vi "RT Config - Dual RT Sweep.vi"(8 "error in (no error)":errorcluster, 11 "1553 Unit Test in":refnum<class "Remote Terminal.lvclass">) -> (0 "error out":errorcluster, 3 "1553 Unit Test out":refnum<class "Remote Terminal.lvclass">)   [LabVIEW 2020, in "Unit Tests.lvlib" / "Remote Terminal.lvclass"]
uses:
  Remote Terminal.lvclass
  Remote Terminal.lvclass/Remote Terminal.ctl
  Remote Terminal/TypeDefs/RT Command Config.ctl
  Frames & Messages/TypeDefs/Command Type.ctl
  Frames & Messages/TypeDefs/Command SubAddress.ctl
  Frames & Messages/TypeDefs/Command Word Count.ctl
  Frames & Messages/TypeDefs/Simplified Parameter Data Table.ctl
  Frames & Messages/TypeDefs/Scaling Information.ctl
  Remote Terminal/TypeDefs/RT Configuration.ctl
  Remote Terminal/TypeDefs/RT-RT Timeout.ctl
  Remote Terminal/TypeDefs/Mode Code 17 Sync Configuration.ctl
  Remote Terminal/TypeDefs/RT Timetag Configuration.ctl
  Remote Terminal/Remote Terminal.lvclass
  C:/Users/MattJ/Desktop/git/bci-1553-labview-api/src/1553 SubComponent/1553 SubComponent.lvclass
  1553 Session/1553 Session.lvclass
  1553 Component/1553 Component.lvclass
  <vilib>/addons/_JKI Toolkits/Caraya/classes/Test/Test.lvclass
  BCI-1553 API.lvlib
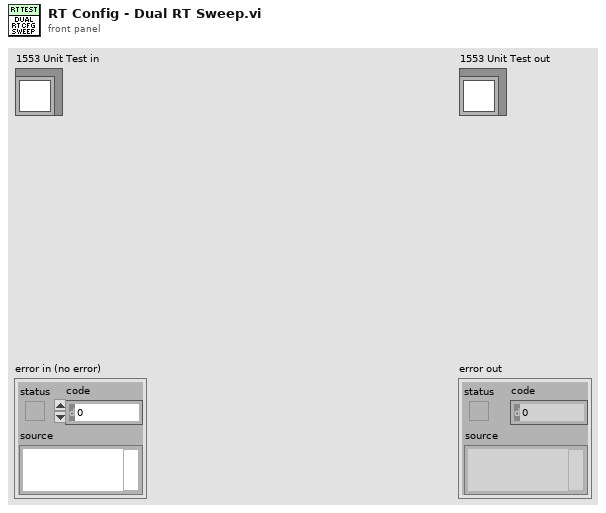
[diagram p1: front panel]
types:
  T1 = typedef "BCI-1553 API.lvlib/Simplified Parameter Data Table.ctl" = cluster{"Parameter Name":string, "Base Word":u16, "Scaling Info":T2}
  T2 = typedef "BCI-1553 API.lvlib/Scaling Information.ctl" = cluster{"Bit Offset":i32, "Bit Count":i32, "LSB Resolution":dbl, "2's Complement":bool, "Big Endian":bool, "Sign Bit":bool}
  T3 = typedef "BCI-1553 API.lvlib/Command SubAddress.ctl" = enum16{"Mode Code", "1", "2", "3", "4", "5", "6", "7", "8", "9", "10", "11", "12", "13", "14", "15", "16", "17", "18", "19", "20", "21", "22", "23", "24", "25", "26", "27", "28", "29", "30"}
  T4 = typedef "BCI-1553 API.lvlib/Command Type.ctl" = enum16{"Transmit", "Receive"}
  T5 = typedef "BCI-1553 API.lvlib/Remote Terminal.lvclass/RT Command Config.ctl" = cluster{"Command Type":T4, "SubAddress":T3, "Word Count\\Mode Code":T6, "Initial Data":u16[], "Data Fields":T1[]}
  T6 = typedef "BCI-1553 API.lvlib/Command Word Count.ctl" = enum16{"1", "2", "3", "4", "5", "6", "7", "8", "9", "10", "11", "12", "13", "14", "15", "16", "17", "18", "19", "20", "21", "22", "23", "24", "25", "26", "27", "28", "29", "30", "31", "32"}
  T7 = typedef "BCI-1553 API.lvlib/Remote Terminal.lvclass/RT Configuration.ctl" = cluster{"RT-RT Timeout":T8, "Inhibit Bus A":bool, "Inhibit Bus B":bool, "Broadcast CMD Invalid":bool, "UnDef MCs Invalid":bool, "Notice 2 Data Storage":bool, "SMCP":bool, "Temp RX Buffer":bool, "Alt BIT Enable":bool, "Auto Bus Shutdown":bool, "MC 16 SR Reset":bool, "MC 17 Sync":T9, "MC 8 Reset":bool, "Remote Terminal Timetag Config":T10}
  T8 = typedef "BCI-1553 API.lvlib/Remote Terminal.lvclass/RT-RT Timeout.ctl" = enum16{"57us", "62us", "100us", "180us"}
  T9 = typedef "BCI-1553 API.lvlib/Remote Terminal.lvclass/Mode Code 17 Sync Configuration.ctl" = enum16{"Sync if Bit 0 = 1", "Sync if Bit 0 = 0", "Sync Unconditionally"}
  T10 = typedef "BCI-1553 API.lvlib/Remote Terminal.lvclass/RT Timetag Configuration.ctl" = enum16{"Disabled", "2us", "4us", "8us", "16us", "32us", "64us"}
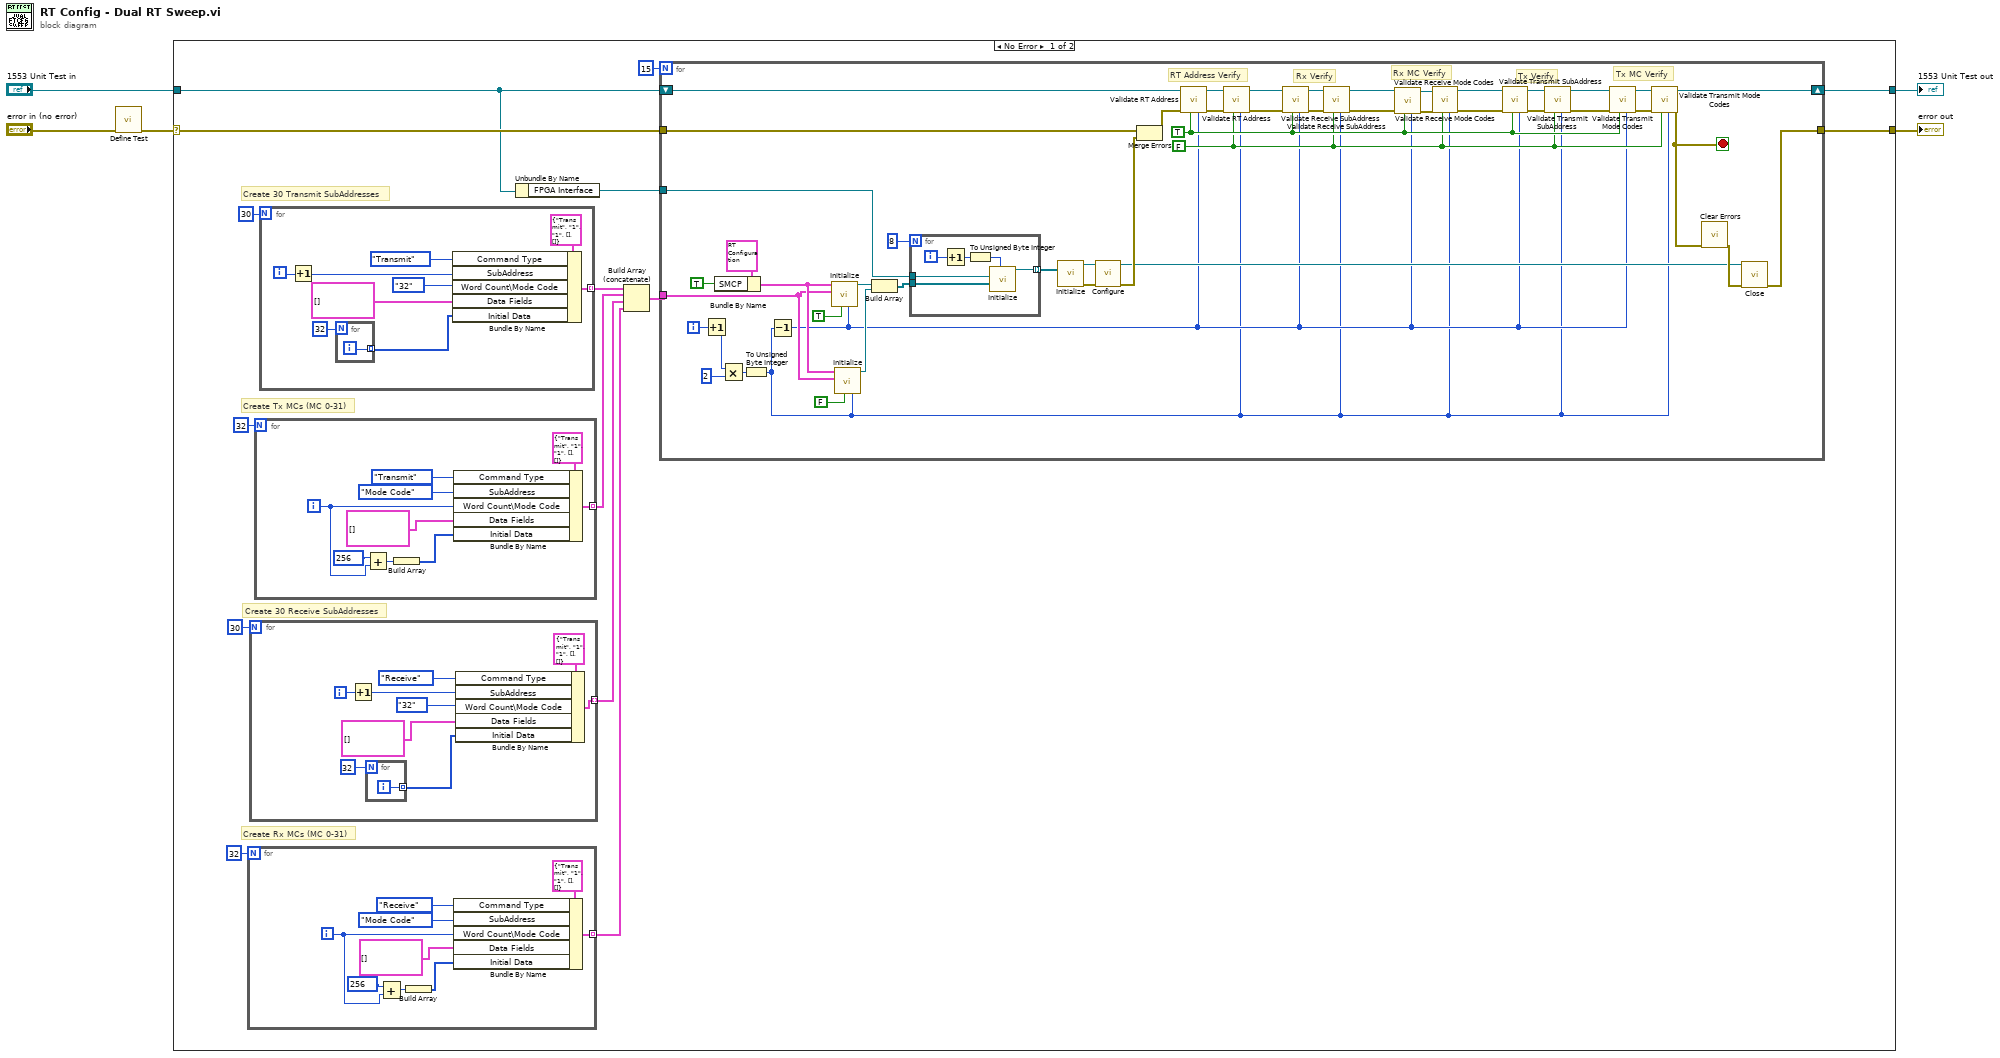
[diagram p0: block diagram]
diagram:
  n1 = call <vilib>:"Define Test.vi"("error in (no error)"="error in (no error)") -> ("error out"=w1:errorcluster)  [unwired: 9 in, 1 out]
  n2 = case shown="No Error" w1 {
    selector: w1 -> [w17 w115]
    tunnel: [w18 w115] -> w5
    tunnel: [w19 w114] -> w3
    tunnel: "1553 Unit Test in" -> [w16 w114]
    frame No Error {
      # "Create Rx MCs (MC 0-31)"
      # "Create Tx MCs (MC 0-31)"
      # "Create 30 Receive SubAddresses"
      # "Create 30 Transmit SubAddresses"
      n3 = for {
        N: 32 -> [_]
        tunnel: [w29] -> w7 mode=indexing
        i -> [w22]
        n4 = Add(x=256, y=w22) -> (x+y=w23:i32)
        n5 = Build Array(w23) -> (w25:i32[])
        n6 = Bundle By Name(cluster=T5 {"Command Type"=enum."Transmit", "SubAddress"=enum."1", "Word Count\\Mode Code"=enum."1", "Initial Data"=[], "Data Fields"=[]} ("RT Commands"), "Command Type"=Command_Type."Receive", "SubAddress"=Command_SubAddress."Mode Code", "Word Count\\Mode Code"=w22, "Data Fields"=T1[] [], "Initial Data"=w25) -> (w29:T5)
      }
      n7 = for {
        N: 30 -> [_]
        tunnel: [w47] -> w9 mode=indexing
        i -> [w42]
        n8 = Increment(x=w42) -> (x+1=w41:i32)
        n9 = for {
          N: 32 -> [_]
          tunnel: [w48] -> w43 mode=indexing
          i -> [w48]
        }
        n10 = Bundle By Name(cluster=T5 {"Command Type"=enum."Transmit", "SubAddress"=enum."1", "Word Count\\Mode Code"=enum."1", "Initial Data"=[], "Data Fields"=[]} ("RT Commands"), "Command Type"=Command_Type."Receive", "SubAddress"=w41, "Word Count\\Mode Code"=Command_Word_Count."32" ("Word Count\\Mode Code"), "Data Fields"=T1[] [], "Initial Data"=w43) -> (w47:T5)
      }
      n11 = for {
        N: 32 -> [_]
        tunnel: [w38] -> w10 mode=indexing
        i -> [w32]
        n12 = Add(x=256, y=w32) -> (x+y=w33:i32)
        n13 = Build Array(w33) -> (w31:i32[])
        n14 = Bundle By Name(cluster=T5 {"Command Type"=enum."Transmit", "SubAddress"=enum."1", "Word Count\\Mode Code"=enum."1", "Initial Data"=[], "Data Fields"=[]} ("RT Commands"), "Command Type"=Command_Type."Transmit", "SubAddress"=Command_SubAddress."Mode Code", "Word Count\\Mode Code"=w32, "Data Fields"=T1[] [], "Initial Data"=w31) -> (w38:T5)
      }
      n15 = for {
        N: 30 -> [_]
        tunnel: [w57] -> w12 mode=indexing
        i -> [w52]
        n16 = Increment(x=w52) -> (x+1=w51:i32)
        n17 = for {
          N: 32 -> [_]
          tunnel: [w58] -> w53 mode=indexing
          i -> [w58]
        }
        n18 = Bundle By Name(cluster=T5 {"Command Type"=enum."Transmit", "SubAddress"=enum."1", "Word Count\\Mode Code"=enum."1", "Initial Data"=[], "Data Fields"=[]} ("RT Commands"), "Command Type"=Command_Type."Transmit", "SubAddress"=w51, "Word Count\\Mode Code"=Command_Word_Count."32" ("Word Count\\Mode Code"), "Data Fields"=T1[] [], "Initial Data"=w53) -> (w57:T5)
      }
      n19 = Unbundle By Name(w16) -> ("FPGA Interface"=w15:refnum<class "FPGA Interface.lvclass">)
      n20 = Build Array (concatenate)(w12, w10, w9, w7) -> (w6:T5[])
      n21 = for {
        N: 15 -> [_]
        shift-right: [w74] -> w19
        shift-left: w16 -> [w97]
        tunnel: [w83] -> w18
        tunnel: w17 -> [w92]
        tunnel: w6 -> [w82]
        tunnel: w15 -> [w81]
        i -> [w104]
        stop <- w70 stop-if-true
        w72 = FALSE ("RT 1?")
        w73 = TRUE ("RT 1?")
        # "Tx MC Verify"
        # "Rx MC Verify"
        # "RT Address Verify"
        # "Rx Verify"
        # "Tx Verify"
        n22 = Increment(x=w104) -> (x+1=w88:i32)
        n23 = Bundle By Name(cluster=T7 {"RT-RT Timeout"=enum."57us", "Inhibit Bus A"=FALSE, "Inhibit Bus B"=FALSE, "Broadcast CMD Invalid"=FALSE, "UnDef MCs Invalid"=FALSE, "Notice 2 Data Storage"=FALSE, "SMCP"=FALSE, "Temp RX Buffer"=FALSE, "Alt BIT Enable"=FALSE, "Auto Bus Shutdown"=FALSE, "MC 16 SR Reset"=FALSE, "MC 17 Sync"=enum."Sync if Bit 0 = 1", "MC 8 Reset"=FALSE, "Remote Terminal Timetag Config"=enum."Disabled"} ("RT Configuration"), "SMCP"=TRUE) -> (w90:T7)
        n24 = Multiply(x=w88, y=2) -> (x*y=w86:i32)
        n25 = To Unsigned Byte Integer(number=w86) -> (unsigned 8bit integer=w69:u8)
        n26 = Decrement(x=w69) -> (x-1=w71:u8)
        n27 = call "Initialize.vi"("Terminal Address"=w71, "RT 1?"=TRUE, "RT Commands"=w82, "RT Configuration"=w90) -> ("Remote Terminal out"=w101:refnum<class "Remote Terminal.lvclass">)  [unwired: 6 in, 1 out]
        n28 = call "Initialize.vi"("Terminal Address"=w69, "RT 1?"=FALSE, "RT Commands"=w82, "RT Configuration"=w90) -> ("Remote Terminal out"=w91:refnum<class "Remote Terminal.lvclass">)  [unwired: 6 in, 1 out]
        n29 = Build Array(w101, w91) -> (w103:refnum<class "Remote Terminal.lvclass">[])
        n30 = for {
          N: 8 -> [_]
          tunnel: [w111] -> w100 mode=indexing
          tunnel: w103 -> [w110]
          tunnel: w81 -> [w109]
          i -> [w113]
          n31 = Increment(x=w113) -> (x+1=w108:i32)
          n32 = To Unsigned Byte Integer(number=w108) -> (unsigned 8bit integer=w112:u8)
          n33 = call "Initialize.vi"("Component ID (1-8)"=w112, "SubComponents"=w110, "FPGA Interface"=w109) -> ("1553 Component out"=w111:refnum<class "1553 Component.lvclass">)  [unwired: 7 in, 1 out]
        }
        n34 = call "Initialize.vi"("Components"=w100) -> ("error out"=w98:errorcluster, "1553 Board out"=w99:refnum<class "1553 Session.lvclass">)  [unwired: 9 in]
        n35 = call-dynamic "Configure.vi"("error in (no error)"=w98, "1553 Board in"=w99) -> ("error out"=w95:errorcluster, "1553 Board out"=w93:refnum<class "1553 Session.lvclass">)  [unwired: 8 in]
        n36 = Merge Errors(w92, w95) -> (w96:errorcluster)
        n37 = call "Validate RT Address.vi"("RT Address (0-30)"=w71, "RT 1?"=w73, "error in (no error)"=w96, "Remote Terminal in"=w97) -> ("error out"=w60:errorcluster, "Remote Terminal out"=w59:refnum<class "Remote Terminal.lvclass">)  [unwired: 6 in]
        n38 = call "Validate RT Address.vi"("RT Address (0-30)"=w69, "RT 1?"=w72, "error in (no error)"=w60, "Remote Terminal in"=w59) -> ("error out"=w85:errorcluster, "Remote Terminal out"=w84:refnum<class "Remote Terminal.lvclass">)  [unwired: 6 in]
        n39 = call "Validate Receive SubAddress.vi"("RT Address (0-30)"=w71, "RT 1?"=w73, "error in (no error)"=w85, "1553 Unit Test in"=w84) -> ("error out"=w62:errorcluster, "1553 Unit Test out"=w61:refnum<class "Remote Terminal.lvclass">)  [unwired: 6 in]
        n40 = call "Validate Receive SubAddress.vi"("RT Address (0-30)"=w69, "RT 1?"=w72, "error in (no error)"=w62, "1553 Unit Test in"=w61) -> ("error out"=w79:errorcluster, "1553 Unit Test out"=w80:refnum<class "Remote Terminal.lvclass">)  [unwired: 6 in]
        n41 = call "Validate Receive Mode Codes.vi"("RT Address (0-30)"=w71, "RT 1?"=w73, "error in (no error)"=w79, "1553 Unit Test in"=w80) -> ("error out"=w64:errorcluster, "1553 Unit Test out"=w63:refnum<class "Remote Terminal.lvclass">)  [unwired: 6 in]
        n42 = call "Validate Receive Mode Codes.vi"("RT Address (0-30)"=w69, "RT 1?"=w72, "error in (no error)"=w64, "1553 Unit Test in"=w63) -> ("error out"=w77:errorcluster, "1553 Unit Test out"=w78:refnum<class "Remote Terminal.lvclass">)  [unwired: 6 in]
        n43 = call "Validate Transmit SubAddress.vi"("RT Address (0-30)"=w71, "RT 1?"=w73, "error in (no error)"=w77, "1553 Unit Test in"=w78) -> ("error out"=w66:errorcluster, "1553 Unit Test out"=w65:refnum<class "Remote Terminal.lvclass">)  [unwired: 6 in]
        n44 = call "Validate Transmit SubAddress.vi"("RT Address (0-30)"=w69, "RT 1?"=w72, "error in (no error)"=w66, "1553 Unit Test in"=w65) -> ("error out"=w75:errorcluster, "1553 Unit Test out"=w76:refnum<class "Remote Terminal.lvclass">)  [unwired: 6 in]
        n45 = call "Validate Transmit Mode Codes.vi"("RT Address (0-30)"=w71, "RT 1?"=w73, "error in (no error)"=w75, "1553 Unit Test in"=w76) -> ("error out"=w67:errorcluster, "1553 Unit Test out"=w68:refnum<class "Remote Terminal.lvclass">)  [unwired: 6 in]
        n46 = call "Validate Transmit Mode Codes.vi"("RT Address (0-30)"=w69, "RT 1?"=w72, "error in (no error)"=w67, "1553 Unit Test in"=w68) -> ("error out"=w70:errorcluster, "1553 Unit Test out"=w74:refnum<class "Remote Terminal.lvclass">)  [unwired: 6 in]
        n47 = call <vilib>:"Clear Errors.vi"("error in (no error)"=w70) -> ("error out"=w94:errorcluster)  [unwired: 5 in, 1 out]
        n48 = call-dynamic "Close.vi"("error in (no error)"=w94, "1553 Board in"=w93) -> ("error out"=w83:errorcluster)  [unwired: 9 in]
      }
    }
    frame Error {
    }
  }
  "error out" <- w5
  "1553 Unit Test out" <- w3
